vi "CAN BOOT Init.vi"(5 "BaudRate":i32, 6 "IDType":u8, 7 "ReceiveDataID":u32, 9 "SendDataID":u32, 10 "CANIndex":i32, 11 "DevHandle":i32) -> (3 "function return":i32)   [LabVIEW 2010, in "can_bootloader.lvlib"]
doc: "int WINAPI CAN_BOOT_Init(int DevHandle,int CANIndex,unsigned int SendDataID,unsigned int ReceiveDataID,unsigned char IDType,int BaudRate);"
uses:
  can_bootloader.lvlib
  USB2XXX/trunk/USB2XXX/USB2XXX/vs2010/Release/USB2XXX.dll
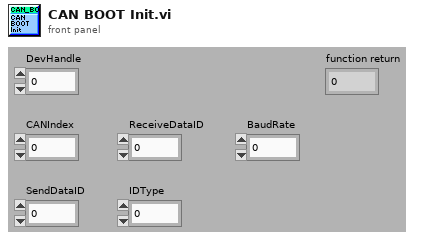
[diagram p1: front panel]
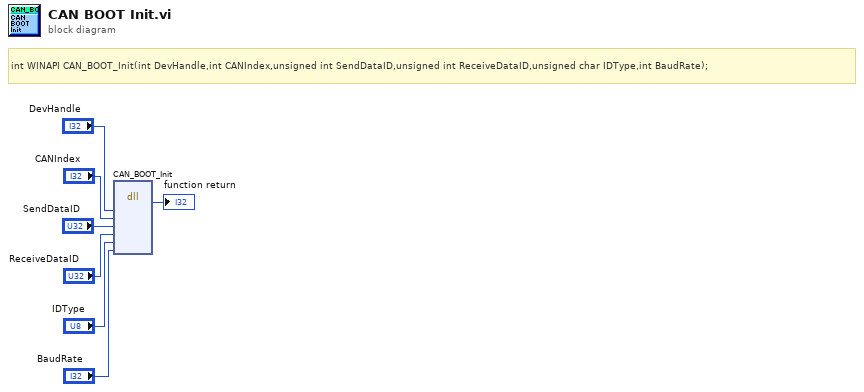
[diagram p0: block diagram]
diagram:
  # "int WINAPI CAN_BOOT_Init(int DevHandle,int CANIndex,unsigned int SendDataID,unsigned int ReceiveDataID,unsigned char IDType,int BaudRate);"
  n1 = dll-call lib="E:/OtherWork/STM32/USB2XXX/trunk/USB2XXX/USB2XXX/vs2010/Release/USB2XXX.*" fn="CAN_BOOT_Init"("DevHandle"="DevHandle", "CANIndex"="CANIndex", "SendDataID"="SendDataID", "ReceiveDataID"="ReceiveDataID", "IDType"="IDType", "BaudRate"="BaudRate") -> (→"function return":i32)  [unwired: 9 in, 2 out]
